vi "XY.vi"(7 "Enable":bool=TRUE, 8 "error in (no error)":errorcluster, 9 "Reset":bool, 10 "Y Input":dynamicdata(graph), 11 "X Input":dynamicdata(graph)) -> (0 "error out":errorcluster, 2 "XY Graph":cluster{"Y":dbl[], "Y":dbl[]}[](graph))   [LabVIEW 2013]
doc: "formats the data displayed on an X-Y Graph.\n--------------------\n\nThis Express VI is configured as follows:\n\nClear data on each call: Off"
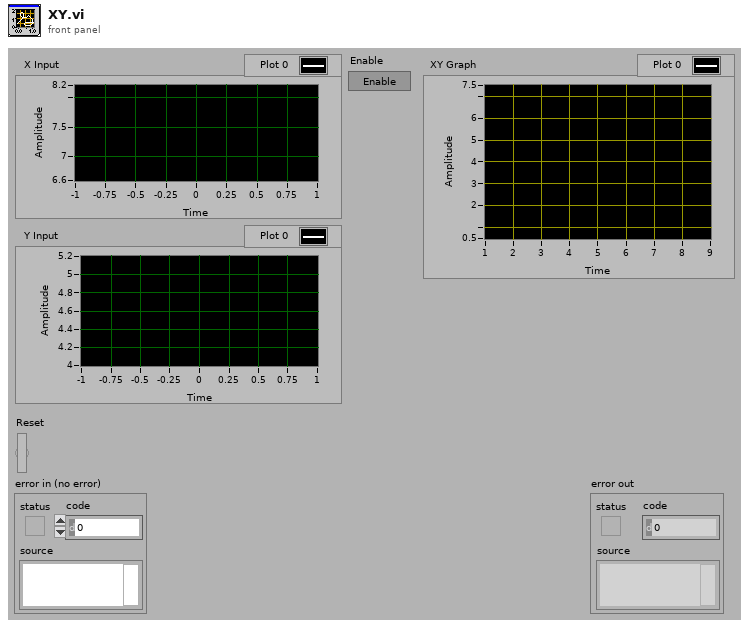
[diagram p1: front panel]
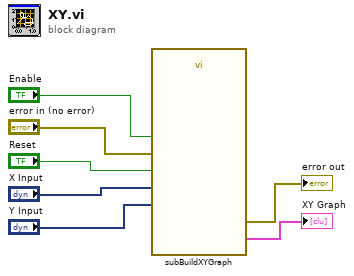
[diagram p0: block diagram]
diagram:
  n1 = call <vilib>:"subBuildXYGraph.vi"("Enable"="Enable", "error in (no error)"="error in (no error)", "Reset"="Reset", "Y Input"="Y Input", "X Input"="X Input") -> ("error out"=→"error out":errorcluster, "XY Graph"=→"XY Graph":cluster{"X":dbl[], "Y":dbl[]}[])  [unwired: 5 in]
